vi "FEM-03 Test.vi"() -> ()   [LabVIEW 2010, in "FEM-03.lvlib"]
uses:
  FEM-03.lvlib
panel:
  in  "Averages":i32=1
  out "Read Rate (ms)":u32=13
  out "GPM (Average)":dbl
  out "error out":errorcluster={"status"=FALSE, "code"=1073676294, "source"="VISA Read in FEM-03.lvlib:Read VAR.vi->FEM-03.lvlib:Read Rate A (GPM).vi->FEM-03.lvlib:FEM-03 Test.vi"}
  in  "VISA resource name":refnum<visa-resource-name>="COM1"
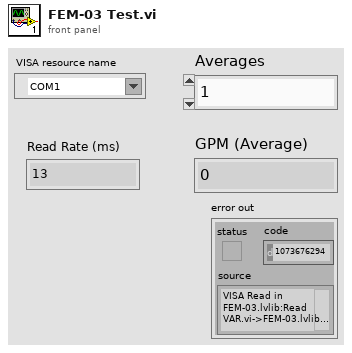
[diagram p1: front panel]
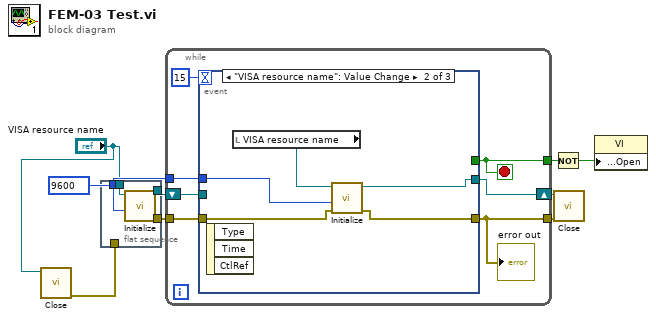
[diagram p0: block diagram]
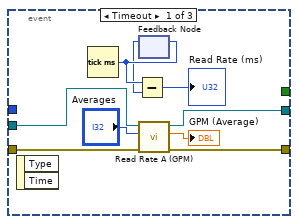
[diagram p2: hidden frame]
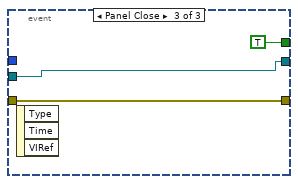
[diagram p3: hidden frame]
diagram:
  w3 = u32 9600 items=["9600"=9600, "38400"=38400, "57600"=57600, "19200"=19200] ("Baud Rate")
  n1 = call "Close.vi"("VISA resource name"="VISA resource name") -> ("error out"=w1:errorcluster)  [unwired: 10 in]
  n2 = flat-sequence {
    tunnel: [w13] -> w9
    tunnel: [w12] -> w8
    tunnel: w3 -> [w11]
    tunnel: "VISA resource name" -> [w10]
    tunnel: w1 -> [_]
    frame #0 {
      n3 = call "Initialize.vi"("Baud Rate"=w11, "VISA resource name"=w10) -> ("error out"=w13:errorcluster, "VISA resource name out"=w12:refnum<visa-resource-name>)  [unwired: 8 in]
    }
  }
  n4 = while {
    tunnel: [w17] -> w5
    shift-right: [w18] -> w6
    shift-left: w8 -> [w19]
    tunnel: w3 -> [w14]
    tunnel: w9 -> [w20]
    tunnel: [w15] -> w7
    stop <- w17 stop-if-true
    n5 = event shown="[1] \"VISA resource name\": Value Change" {
      selector: _ -> [_ _ _]
      dyn-events: _ -> [_ _ _]
      timeout: 15 -> [_ _ _]
      tunnel: w20 -> [w29 w33 w36]
      tunnel: w19 -> [w28 _ w35]
      tunnel: [_ _ TRUE ("stop")] -> w17
      tunnel: [w27 w34 w36] -> w15
      tunnel: [w26 w30 w35] -> w18
      tunnel: w14 -> [_ w31 _]
      event Timeout {
        n6 = event-data() -> ()  [unwired: 1 in, 2 out]
        n7 = Tick Count (ms)() -> (millisecond timer value=w24:u32)
        n8 = feedback #1() -> (w23:u32)  [unwired: 1 in]
        n9 = Subtract(x=w24, y=w23) -> (x-y=→"Read Rate (ms)":u32)
        n10 = feedback-in #1(w24) -> ()
        n11 = call "Read Rate A (GPM).vi"("error out"=w29, "Averages"="Averages", "VISA resource name out"=w28) -> ("error IO"=w27:errorcluster, "GPM"=→"GPM (Average)":dbl, "VISA resource  out"=w26:refnum<visa-resource-name>)  [unwired: 6 in]
      }
      event "VISA resource name": Value Change {
        n12 = event-data() -> ()  [unwired: 1 in, 3 out]
        n13 = local read "VISA resource name"() -> (w32:refnum<visa-resource-name>)
        n14 = call "Initialize.vi"("error in (no error)"=w33, "Baud Rate"=w31, "VISA resource name"=w32) -> ("error out"=w34:errorcluster, "VISA resource name out"=w30:refnum<visa-resource-name>)  [unwired: 7 in]
      }
      event Panel Close {
        n15 = event-data() -> ()  [unwired: 1 in, 3 out]
      }
    }
    "error out" <- w15
  }
  n16 = Not(x=w5) -> (.not. x?=w4:bool)
  n17 = call "Close.vi"("error in (no error)"=w7, "VISA resource name"=w6) -> ()  [unwired: 9 in, 1 out]
  n18 = property class="VI"("Front Panel.Open"=w4) -> ()  [unwired: 2 in, 2 out]
